vi "eventHandler.vi"(8 "error in (no error)":errorcluster, 9 ":HWControllerEvents":refnum<class "HWControllerEvents.lvclass">, 10 "ExperimentControlEvents":refnum<class "ExperimentControlEvents.lvclass">, 11 "ExperimentControl in":refnum<class "ExperimentControl.lvclass">) -> (0 "error out":errorcluster, 3 "ExperimentControl out":refnum<class "ExperimentControl.lvclass">)   [LabVIEW 2011, in "Views.lvlib" / "ExperimentControl.lvlib" / "ExperimentControl.lvclass"]
uses:
  ExperimentControl.lvclass
  Events/ExperimentControlEvents.lvclass
  Hal/HWController/HWControllerEvents/HWControllerEvents.lvclass
  ExperimentControl.lvclass/ExperimentControl.ctl
  Events/Event.lvclass
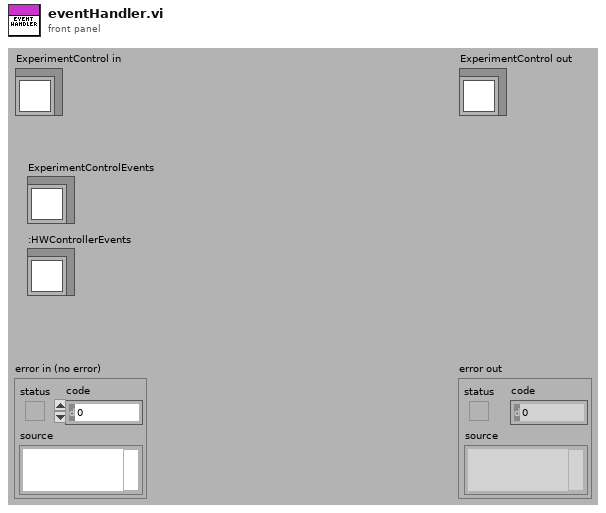
[diagram p1: front panel]
types:
  T1 = enum16{"Ready", "Compiling", "Configured", "Running", "Stopping", "Unresolved Error"}
  T2 = enum16{"close", "stopRunning", "runSingleScript", "runExperiment", "runExperimentScript", "Unregistered", "hasStopped"}
  T3 = cluster{"Array":path[], "Enum":enum16{"runListOnce", "loopOverList"}}
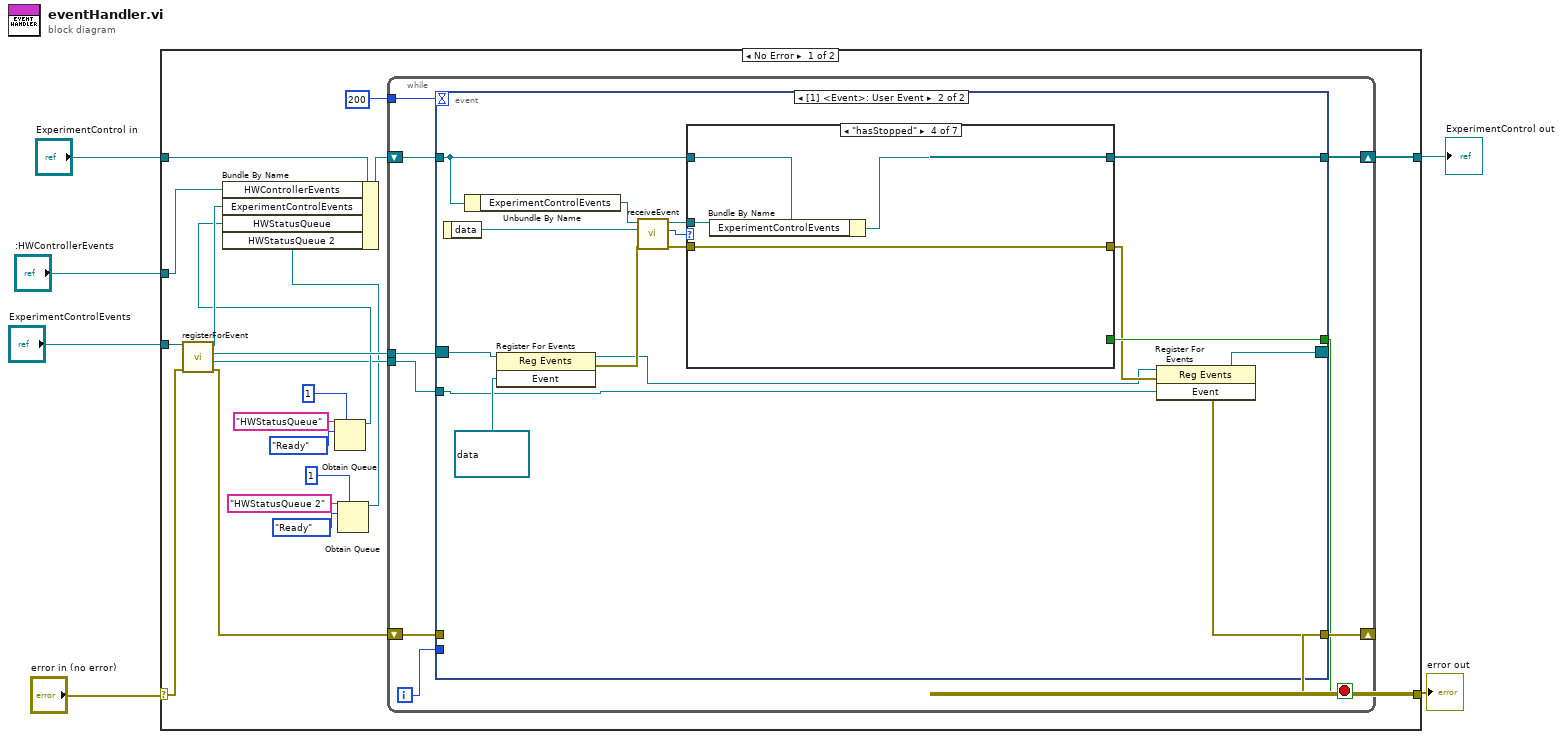
[diagram p0: block diagram]
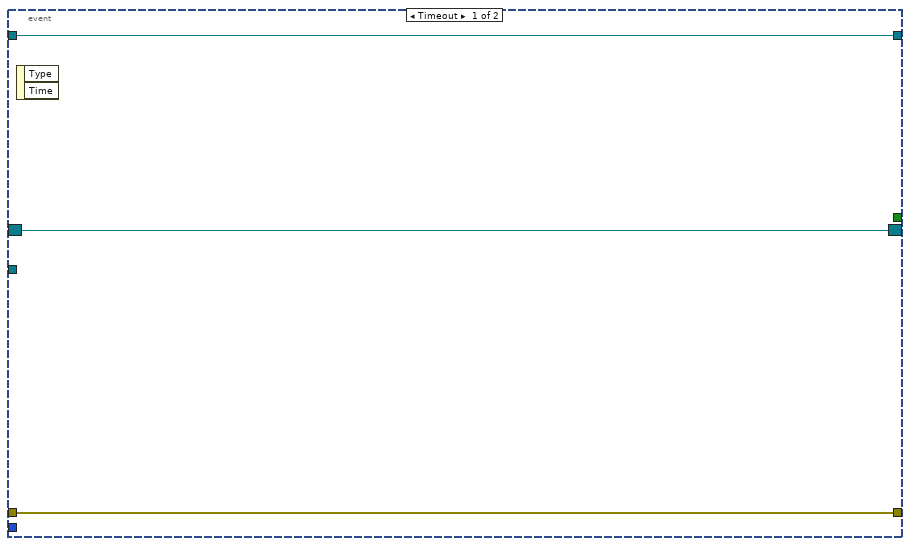
[diagram p2: hidden frame]
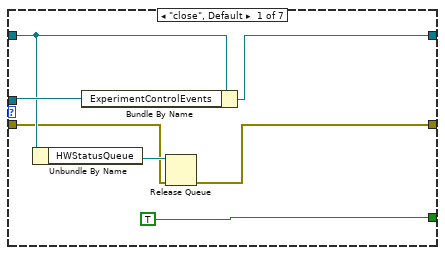
[diagram p3: hidden frame]
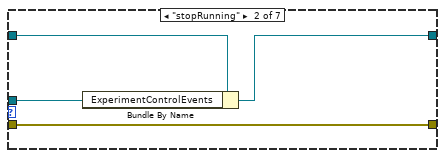
[diagram p4: hidden frame]
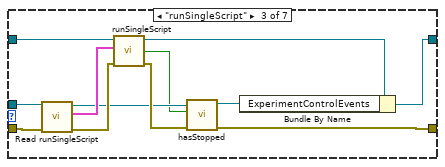
[diagram p5: hidden frame]
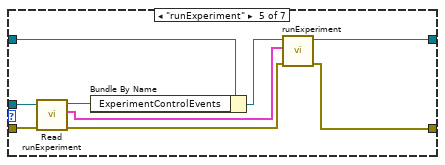
[diagram p6: hidden frame]
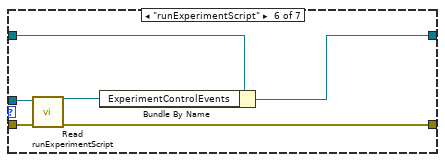
[diagram p7: hidden frame]
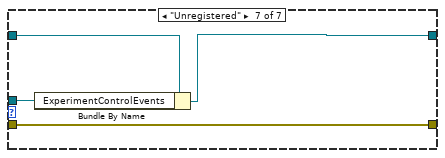
[diagram p8: hidden frame]
diagram:
  n1 = case shown="No Error" "error in (no error)" {
    selector: "error in (no error)" -> [w21 w102]
    tunnel: [w25 w102] -> w5
    tunnel: [w26 w101] -> w1
    tunnel: "ExperimentControl in" -> [w24 w101]
    tunnel: "ExperimentControlEvents" -> [w22 _]
    tunnel: ":HWControllerEvents" -> [w17 _]
    frame No Error {
      n2 = call "registerForEvent.vi"("error in (no error)"=w21, "Event in"=w22) -> ("error out"=w19:errorcluster, "Event"=w11:refnum<user-event>, "Event Registration Refnum"=w20:refnum<event-registration>, "Event out"=w18:refnum<class "ExperimentControlEvents.lvclass">)  [unwired: 6 in]
      n3 = Obtain Queue(max queue size (-1, unlimited)=1, name (unnamed)="HWStatusQueue", element data type=T1."Ready" ("status")) -> (queue out=w12:refnum<queue>)  [unwired: 2 in, 2 out]
      n4 = Obtain Queue(max queue size (-1, unlimited)=1, name (unnamed)="HWStatusQueue 2", element data type=T1."Ready" ("status")) -> (queue out=w7:refnum<queue>)  [unwired: 2 in, 2 out]
      n5 = Bundle By Name(cluster=w24, "HWControllerEvents"=w17, "ExperimentControlEvents"=w18, "HWStatusQueue"=w12, "HWStatusQueue 2"=w7) -> (w23:refnum<class "ExperimentControl.lvclass">)
      n6 = while {
        shift-right: [w32] -> w25
        shift-left: w19 -> [w33]
        shift-right: [w35] -> w26
        shift-left: w23 -> [w34]
        tunnel: w20 -> [w31]
        tunnel: 200 -> [w27]
        tunnel: w11 -> [w28]
        i -> [w29]
        stop <- w30 stop-if-true
        n7 = event shown="[1] <Event>: User Event" {
          selector: w31 -> [w36 w43]
          dyn-events: [w36 w45] -> _
          timeout: w27 -> [_ _]
          tunnel: [w38 w47] -> w35
          tunnel: w34 -> [w38 w49]
          tunnel: w33 -> [w37 _]
          tunnel: [w37 w44] -> w32
          tunnel: [_ w51] -> w30
          tunnel: w29 -> [_ _]
          tunnel: w28 -> [_ w39]
          event Timeout {
            n8 = event-data() -> ()  [unwired: 1 in, 2 out]
          }
          event User Event {
            n9 = event-data() -> ("data"=w53:refnum<class>)  [unwired: 1 in]
            n10 = Unbundle By Name(w49) -> ("ExperimentControlEvents"=w54:refnum<class "ExperimentControlEvents.lvclass">)
            n11 = register-events(reference=w43, refnum<user-event> refnum ("Event")) -> (reference out=w40:refnum<event-registration>, error out=w41:errorcluster)  [unwired: 1 in]
            n12 = call "receiveEvent.vi"("error in (no error)"=w41, "data"=w53, "ExperimentControlEvents in"=w54) -> ("error out"=w50:errorcluster, "Enum"=w52:T2, "ExperimentControlEvents out"=w48:refnum<class "ExperimentControlEvents.lvclass">)  [unwired: 6 in]
            n13 = case shown="\"hasStopped\"" w52 {
              tunnel: w48 -> [w59 w63 w75 w80 w90 w93 w99]
              tunnel: [TRUE _ _ _ _ _ _] -> w51
              tunnel: w50 -> [w56 w62 w74 w81 w89 w94 w100]
              tunnel: [w55 w62 w73 w81 w83 w91 w100] -> w46
              tunnel: w49 -> [w58 w65 w71 w79 w87 w96 w98]
              tunnel: [w60 w64 w67 w78 w85 w95 w97] -> w47
              frame "close", Default {
                n14 = Unbundle By Name(w58) -> ("HWStatusQueue"=w57:refnum<queue>)
                n15 = Bundle By Name(cluster=w58, "ExperimentControlEvents"=w59) -> (w60:refnum<class "ExperimentControl.lvclass">)
                n16 = Release Queue(queue=w57, error in (no error)=w56) -> (error out=w55:errorcluster)  [unwired: 1 in, 2 out]
              }
              frame "stopRunning" {
                n17 = Bundle By Name(cluster=w65, "ExperimentControlEvents"=w63) -> (w64:refnum<class "ExperimentControl.lvclass">)
              }
              frame "runSingleScript" {
                n18 = call "Read runSingleScript.vi"("error in (no error)"=w74, "ExperimentControlEvents in"=w75) -> ("error out"=w77:errorcluster, "runSingleScript"=w76:cluster{"Path":path, "HWLoop":bool}, "ExperimentControlEvents out"=w70:refnum<class "ExperimentControlEvents.lvclass">)  [unwired: 7 in]
                n19 = call "runSingleScript.vi"("error in (no error)"=w77, "runSingleScript"=w76, "ExperimentControl in"=w71) -> ("error out"=w72:errorcluster, "stoppedByUser"=w66:bool, "ExperimentControl out"=w68:refnum<class "ExperimentControl.lvclass">)  [unwired: 5 in, 1 out]
                n20 = call "hasStopped.vi"("error in (no error)"=w72, "stoppedByUser"=w66, "ExperimentControlEvents in"=w70) -> ("error out"=w73:errorcluster, "ExperimentControlEvents out"=w69:refnum<class "ExperimentControlEvents.lvclass">)  [unwired: 7 in]
                n21 = Bundle By Name(cluster=w68, "ExperimentControlEvents"=w69) -> (w67:refnum<class "ExperimentControl.lvclass">)
              }
              frame "hasStopped" {
                n22 = Bundle By Name(cluster=w79, "ExperimentControlEvents"=w80) -> (w78:refnum<class "ExperimentControl.lvclass">)
              }
              frame "runExperiment" {
                n23 = call "Read runExperiment.vi"("error in (no error)"=w89, "ExperimentControlEvents in"=w90) -> ("error out"=w84:errorcluster, "runExperiment"=w82:T3, "ExperimentControlEvents out"=w88:refnum<class "ExperimentControlEvents.lvclass">)  [unwired: 7 in]
                n24 = Bundle By Name(cluster=w87, "ExperimentControlEvents"=w88) -> (w86:refnum<class "ExperimentControl.lvclass">)
                n25 = call "runExperiment.vi"("error in (no error)"=w84, "runExperiment"=w82, "ExperimentControl in"=w86) -> ("error out"=w83:errorcluster, "ExperimentControl out"=w85:refnum<class "ExperimentControl.lvclass">)  [unwired: 7 in]
              }
              frame "runExperimentScript" {
                n26 = call "Read runExperimentScript.vi"("error in (no error)"=w94, "ExperimentControlEvents in"=w93) -> ("error out"=w91:errorcluster, "ExperimentControlEvents out"=w92:refnum<class "ExperimentControlEvents.lvclass">)  [unwired: 7 in, 1 out]
                n27 = Bundle By Name(cluster=w96, "ExperimentControlEvents"=w92) -> (w95:refnum<class "ExperimentControl.lvclass">)
              }
              frame "Unregistered" {
                n28 = Bundle By Name(cluster=w98, "ExperimentControlEvents"=w99) -> (w97:refnum<class "ExperimentControl.lvclass">)
              }
            }
            n29 = register-events(reference=w40, error in=w46, w39) -> (reference out=w45:refnum<event-registration>, error out=w44:errorcluster)
          }
        }
      }
    }
    frame Error {
    }
  }
  "error out" <- w5
  "ExperimentControl out" <- w1
